vi "IMAQ FPGA Camera Link Line Builder (8 Tap U8 4X-1Y).vi"(8 "Input Valid In":bool=TRUE, 9 "Frame Valid In":bool, 10 "Line Valid In":bool, 11 "Pixel Data In":u8[](array[numeric])=[0, 0, 0, 0, 0, 0, 0, 0]) -> (0 "Output Valid":bool, 1 "Frame Valid Out":bool, 2 "Line Valid Out":bool, 3 "Pixel Bus x8 Out":cluster{"Pixels":u8[], "DV":bool[]}, 5 "Overflow":bool)   [LabVIEW 2017]
doc: "Camera Link cameras may return pixels from different parts of the image on each pixel clock. The Line Builder takes those pixels and combines them over multiple cycles to return a Pixel Bus of 8 pixels that are adjacent to each other. \n\nThis instance expects a camera with eigth taps (i.e. eight pixels returned on each pixel clock). The first two taps represents the left quarter of the image and the first valid pixels from these taps are located on the left of the image (pixels 0 and 1). The next two taps represents the next quarter of the image and the first valid pixels from these tap are located at Width/4, Width/4+1 of the image. The next two taps represents the next quarter of the image and the first valid pixels from these taps is located in the middle of the image (width/2 and width/2+1). The last two taps represent the last quarter of the image and the first valid pixels from these taps is located at 3/4*Width, and 3/4*Width +1 of the image."
uses:
  <vilib>/visionFPGA/Basics/Camera Link Acquisition/Controls/IMAQ FPGA Camera Link Line Builder State.ctl
  <vilib>/rvi/Emulation/niFpgaSctlEmulationGetInTimedLoop.vi
  <vilib>/Utility/error.llb/Clear Errors.vi
  <vilib>/rvi/DataTransferAndStorage/Container/Common/niFpgaContainerGetUniqueNameForEmu.vi
  <vilib>/rvi/DataTransferAndStorage/Container/Common/niFpgaContainerSetEmuInfo.vi
  <vilib>/rvi/eio/common/nirviEmuReportErrorAndStop.vi
  <vilib>/rvi/DataTransferAndStorage/Container/Common/niFpgaContainerExecOnDevCompGetState.vi
  <vilib>/rvi/Emulation/niFpgaEmulationIsFPGAContextNoSignature.vi
  <vilib>/rvi/Emulation/niFpgaProcessEmulError.vi
  <vilib>/rvi/errors/nirviReportUnexpectedCaseInternalError (U32).vi
  <vilib>/rvi/Memory/Memory_Emulation/niFpgaMemoryEmulationCacheClearOnFirstRun.vi
  <vilib>/rvi/Memory/Memory_Emulation/nirvimemoryEmulationManagerCache_MakeExclusive.vi
  <vilib>/rvi/Memory/Memory_Emulation/niFpgaMemoryEmulationValidateCache.vi
  <vilib>/rvi/Memory/Memory_Emulation/nirvimemoryEmulationManagerCache_InsertValue.vi
  <vilib>/rvi/Memory/Memory_Emulation/nirvimemoryEmulationManagerCache_ReleaseExclusive.vi
  <vilib>/rvi/Memory/Memory_Emulation/nirvimemoryEmulationManagerCache_GetValue.vi
  <vilib>/rvi/Memory/Memory_Emulation/nirvimemoryEmulationManagerCache_SetValue.vi
  <vilib>/rvi/Emulation/niFpgaSctlEmulationResourceMgr.vi
  <vilib>/rvi/LocalResourceManager/LocalResourceManager.xnode
  <vilib>/rvi/DataTransferAndStorage/Container/XNode/niFpgaContainer.xnode
  <vilib>/rvi/Memory/Memory_Emulation/niFpgaMemoryEmulationRefIn.vi
  <vilib>/visionFPGA/NI_VDM_FPGA_Basics.lvlib
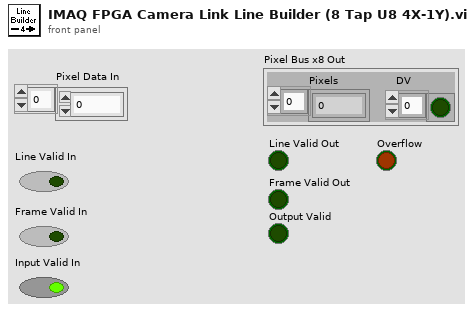
[diagram p1: front panel]
types:
  T1 = typedef "IMAQ FPGA Camera Link Line Builder State.ctl" = enum16{"Wait for First Valid Pixels", "Update Section 1", "Update Section 2", "Update Section 3", "Update Last Section", "Add Final Pack", "Add End of Line", "Check End of Image"}
  T2 = cluster{bool, u16, "Falling Edge":bool, bool, "Falling Edge":bool}
  T3 = cluster{bool, u16, "Falling Edge":bool, "Enum":T1, "Falling Edge":bool}
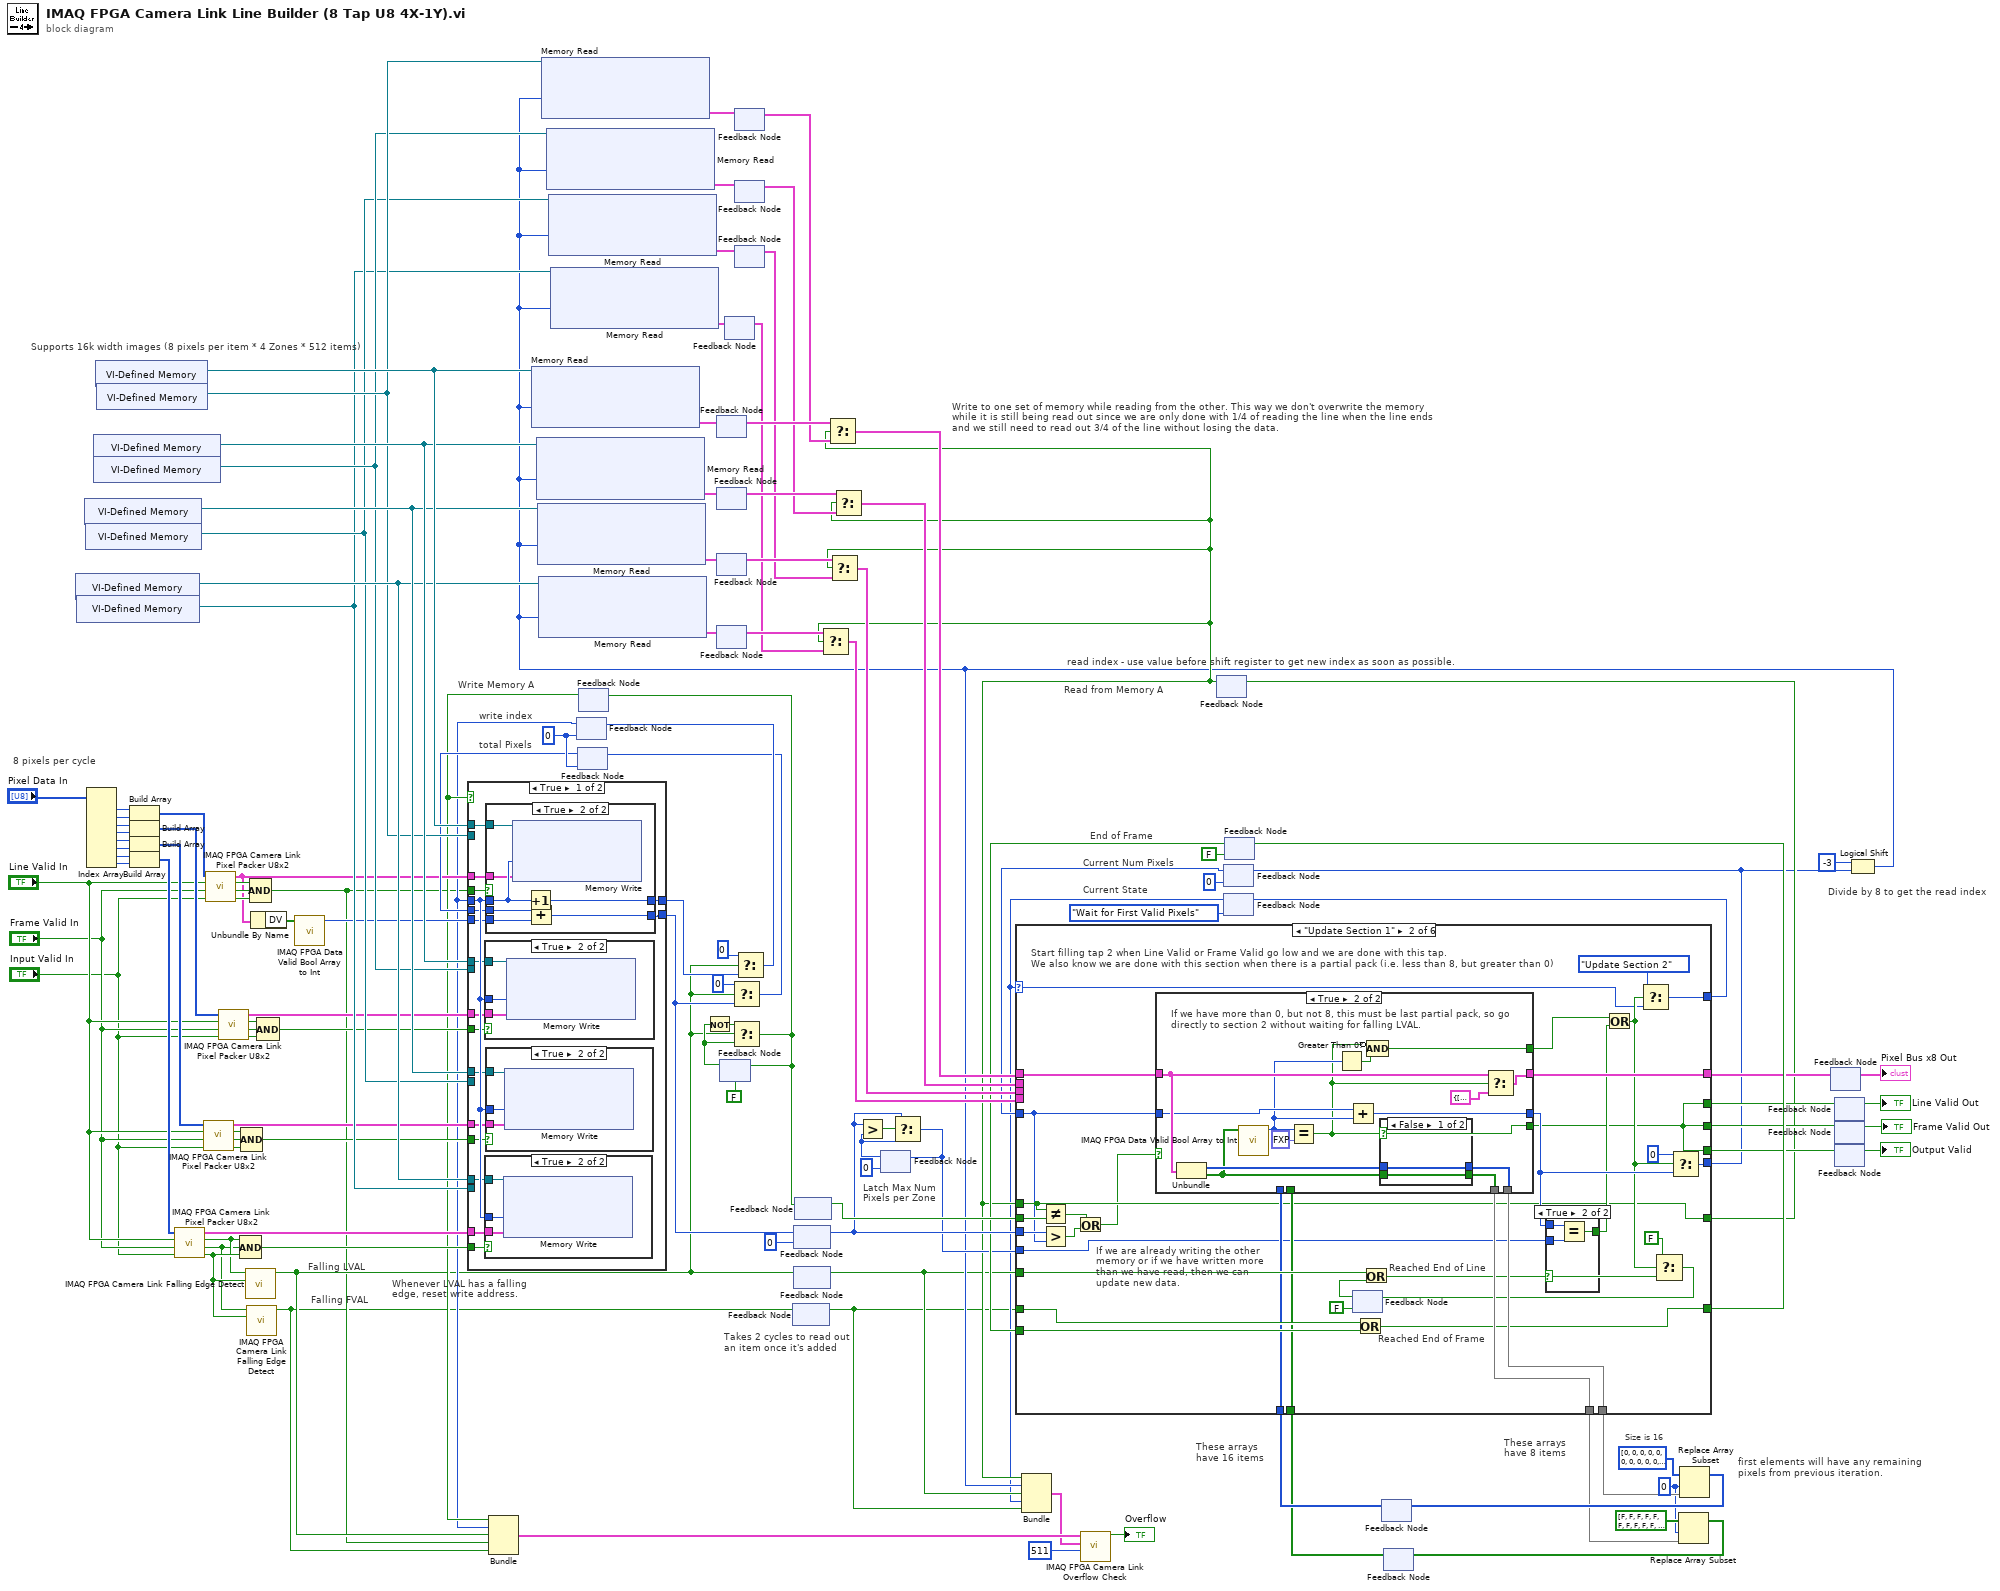
[diagram p0: block diagram]
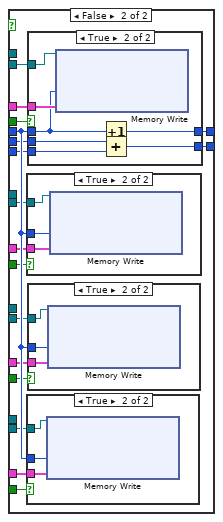
[diagram p6: hidden frame]
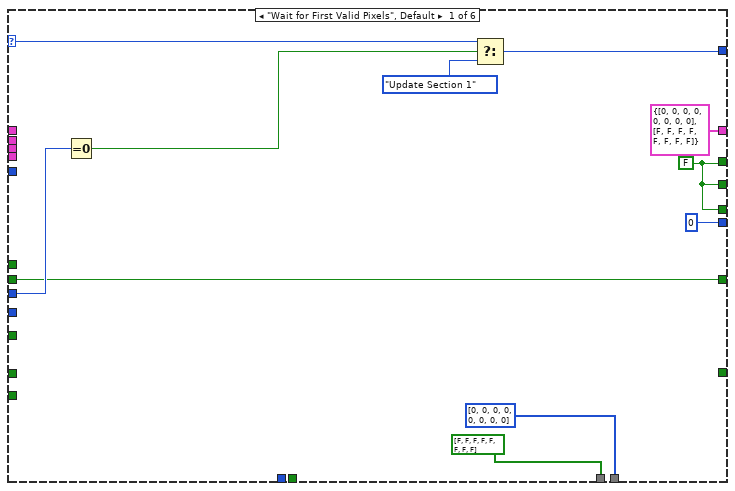
[diagram p11: hidden frame]
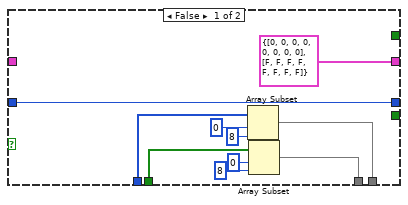
[diagram p12: hidden frame]
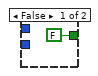
[diagram p14: hidden frame]
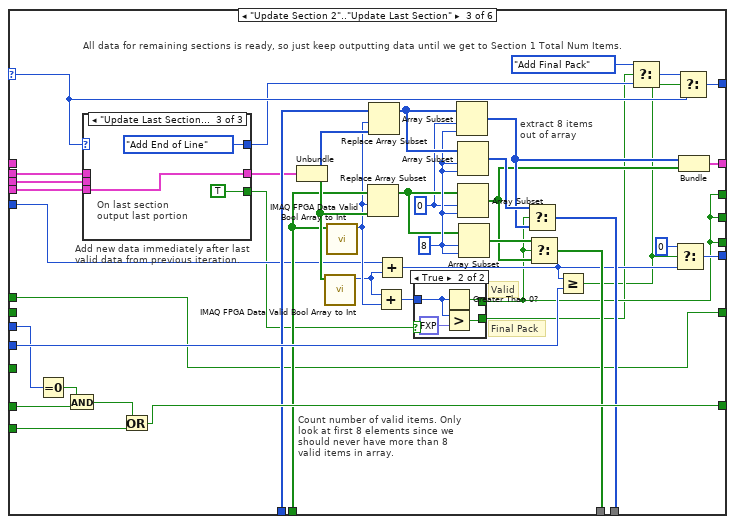
[diagram p15: hidden frame]
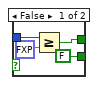
[diagram p16: hidden frame]
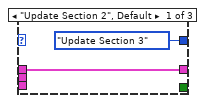
[diagram p17: hidden frame]
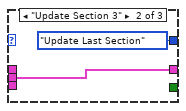
[diagram p18: hidden frame]
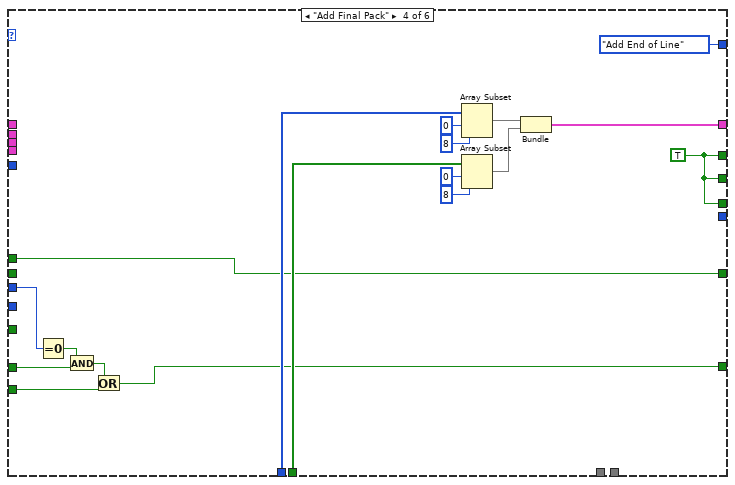
[diagram p19: hidden frame]
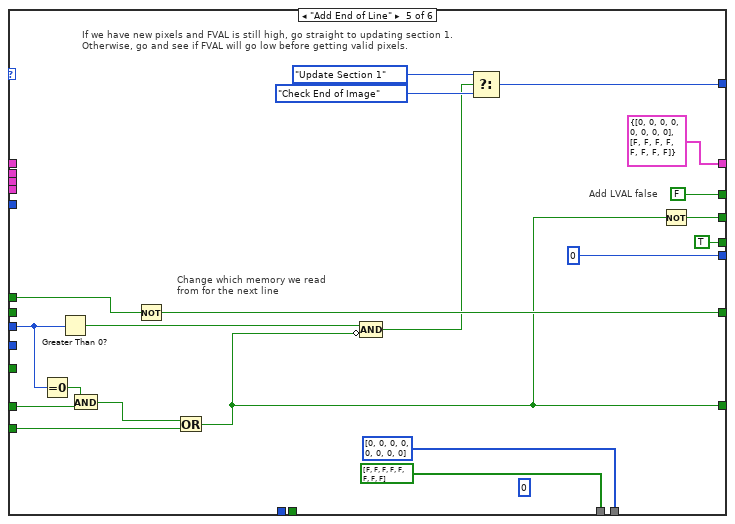
[diagram p20: hidden frame]
diagram:
  w41 = 0 ("index")
  w37 = u16 0
  # "Divide by 8 to get the read index"
  # "Latch Max Num Pixels per Zone"
  # "total Pixels"
  # "These arrays have 8 items"
  # "These arrays have 16 items"
  # "first elements will have any remaining pixels from previous iteration."
  # "Size is 16"
  # "Read from Memory A"
  # "Write Memory A"
  # "Write to one set of memory while reading from the other. This way we don't overwrite the memory while it is still being read out since we are only done with 1/4 of reading the line when the line ends and we still need to read out 3/4 of the line without losing the data."
  # "Falling FVAL"
  # "Falling LVAL"
  # "read index - use value before shift register to get new index as soon as possible."
  # "write index"
  # "Current State"
  # "End of Frame"
  # "Takes 2 cycles to read out an item once it's added"
  # "Current Num Pixels"
  # "Whenever LVAL has a falling edge, reset write address."
  # "Supports 16k width images (8 pixels per item * 4 Zones * 512 items)"
  # "8 pixels per cycle"
  n1 = xnode "VI-Defined Memory"() -> ("Memory Out"=w88:refnum<k21>)
  n2 = xnode "VI-Defined Memory"() -> ("Memory Out"=w80:refnum<k21>)
  n3 = xnode "VI-Defined Memory"() -> ("Memory Out"=w89:refnum<k21>)
  n4 = xnode "VI-Defined Memory"() -> ("Memory Out"=w81:refnum<k21>)
  n5 = Index Array(array="Pixel Data In") -> (element #1=w119:u8, element #2=w118:u8, element #3=w111:u8, element #4=w110:u8, element #5=w108:u8, element #6=w107:u8, element #7=w105:u8, element #8=w104:u8)  [unwired: 8 in]
  n6 = xnode "VI-Defined Memory"() -> ("Memory Out"=w90:refnum<k21>)
  n7 = xnode "VI-Defined Memory"() -> ("Memory Out"=w82:refnum<k21>)
  n8 = xnode "VI-Defined Memory"() -> ("Memory Out"=w91:refnum<k21>)
  n9 = xnode "VI-Defined Memory"() -> ("Memory Out"=w83:refnum<k21>)
  n10 = Build Array(w119, w118) -> (w117:u8[])
  n11 = Build Array(w111, w110) -> (w109:u8[])
  n12 = Build Array(w108, w107) -> (w106:u8[])
  n13 = Build Array(w105, w104) -> (w103:u8[])
  n14 = call <vilib>:"IMAQ FPGA Camera Link Pixel Packer U8x2.vi"("Input Valid"="Input Valid In", "Frame Valid In"="Frame Valid In", "Line Valid In"="Line Valid In", "Pixels In"=w103) -> ("Output Valid"=w30:bool, "Frame Valid Out"=w28:bool, "Line Valid Out"=w29:bool, "Pixel Bus x8 Out"=w65:cluster{"Pixels":u8[], "DV":bool[]})  [unwired: 4 in]
  n15 = call <vilib>:"IMAQ FPGA Camera Link Pixel Packer U8x2.vi"("Input Valid"="Input Valid In", "Frame Valid In"="Frame Valid In", "Line Valid In"="Line Valid In", "Pixels In"=w106) -> ("Output Valid"=w55:bool, "Frame Valid Out"=w56:bool, "Line Valid Out"=w57:bool, "Pixel Bus x8 Out"=w66:cluster{"Pixels":u8[], "DV":bool[]})  [unwired: 4 in]
  n16 = call <vilib>:"IMAQ FPGA Camera Link Pixel Packer U8x2.vi"("Input Valid"="Input Valid In", "Frame Valid In"="Frame Valid In", "Line Valid In"="Line Valid In", "Pixels In"=w117) -> ("Output Valid"=w114:bool, "Frame Valid Out"=w115:bool, "Line Valid Out"=w116:bool, "Pixel Bus x8 Out"=w31:cluster{"Pixels":u8[], "DV":bool[]})  [unwired: 4 in]
  n17 = call <vilib>:"IMAQ FPGA Camera Link Pixel Packer U8x2.vi"("Input Valid"="Input Valid In", "Frame Valid In"="Frame Valid In", "Line Valid In"="Line Valid In", "Pixels In"=w109) -> ("Output Valid"=w61:bool, "Frame Valid Out"=w60:bool, "Line Valid Out"=w59:bool, "Pixel Bus x8 Out"=w67:cluster{"Pixels":u8[], "DV":bool[]})  [unwired: 4 in]
  n18 = Compound Arithmetic op=AND(w29, w28, w30) -> (w53:bool)
  n19 = Compound Arithmetic op=AND(w57, w56, w55) -> (w54:bool)
  n20 = call <vilib>:"IMAQ FPGA Camera Link Falling Edge Detect.vi"("Input Valid"=w30, "Input"=w29) -> ("Falling Edge"=w12:bool)  [unwired: 9 in]
  n21 = call <vilib>:"IMAQ FPGA Camera Link Falling Edge Detect.vi"("Input Valid"=w30, "Input"=w28) -> ("Falling Edge"=w10:bool)  [unwired: 9 in]
  n22 = Compound Arithmetic op=AND(w116, w115, w114) -> (w11:bool)
  n23 = Unbundle By Name(w31) -> ("DV"=w40:bool[])
  n24 = Compound Arithmetic op=AND(w59, w60, w61) -> (w58:bool)
  n25 = call <vilib>:"IMAQ FPGA Data Valid Bool Array to Int.vi"("DV In"=w40) -> ("Sum DV Out"=w35:u8)  [unwired: 10 in]
  n26 = feedback #1(w37) -> (w13:u16)
  n27 = feedback #2(w37) -> (w36:u16)
  n28 = feedback #3() -> (w14:bool)  [unwired: 1 in]
  n29 = case shown="True" w14 {
    tunnel: [w142 w177] -> w120
    tunnel: w13 -> [w141 w176]
    tunnel: w11 -> [w132 w175]
    tunnel: w31 -> [w140 w174]
    tunnel: w67 -> [w139 w173]
    tunnel: w66 -> [w138 w172]
    tunnel: w65 -> [w137 w171]
    tunnel: w91 -> [w136 _]
    tunnel: w90 -> [w135 _]
    tunnel: w89 -> [w134 _]
    tunnel: w88 -> [w133 _]
    tunnel: w83 -> [_ w170]
    tunnel: w82 -> [_ w169]
    tunnel: w81 -> [_ w168]
    tunnel: w80 -> [_ w167]
    tunnel: w58 -> [w131 w166]
    tunnel: w54 -> [w130 w165]
    tunnel: w53 -> [w129 w164]
    tunnel: [w128 w163] -> w34
    tunnel: w36 -> [w127 w162]
    tunnel: w35 -> [w126 w161]
    frame True {
      n30 = case shown="True" w131 {
        tunnel: w139 -> [_ w150]
        tunnel: w135 -> [_ w151]
        tunnel: w141 -> [_ w149]
        frame False {
        }
        frame True {
          n31 = xnode ("Memory Write")("Address"=w149, "Data"=w150, "Memory In"=w151) -> ()  [unwired: 1 out]
        }
      }
      n32 = case shown="True" w129 {
        tunnel: w137 -> [_ w144]
        tunnel: w133 -> [_ w145]
        tunnel: w141 -> [_ w143]
        frame False {
        }
        frame True {
          n33 = xnode ("Memory Write")("Address"=w143, "Data"=w144, "Memory In"=w145) -> ()  [unwired: 1 out]
        }
      }
      n34 = case shown="True" w132 {
        tunnel: [w152 w154] -> w142
        tunnel: w141 -> [w153 w159]
        tunnel: w136 -> [_ w160]
        tunnel: w140 -> [_ w158]
        tunnel: [w153 w157] -> w128
        tunnel: w127 -> [w152 w156]
        tunnel: w126 -> [_ w155]
        frame False {
        }
        frame True {
          n35 = xnode ("Memory Write")("Address"=w159, "Data"=w158, "Memory In"=w160) -> ()  [unwired: 1 out]
          n36 = Increment(x=w159) -> (x+1=w157:u16)
          n37 = Add(x=w156, y=w155) -> (x+y=w154:u16)
        }
      }
      n38 = case shown="True" w130 {
        tunnel: w138 -> [_ w147]
        tunnel: w134 -> [_ w148]
        tunnel: w141 -> [_ w146]
        frame False {
        }
        frame True {
          n39 = xnode ("Memory Write")("Address"=w146, "Data"=w147, "Memory In"=w148) -> ()  [unwired: 1 out]
        }
      }
    }
    frame False {
      n40 = case shown="True" w166 {
        tunnel: w173 -> [_ w185]
        tunnel: w169 -> [_ w186]
        tunnel: w176 -> [_ w184]
        frame False {
        }
        frame True {
          n41 = xnode ("Memory Write")("Address"=w184, "Data"=w185, "Memory In"=w186) -> ()  [unwired: 1 out]
        }
      }
      n42 = case shown="True" w164 {
        tunnel: w171 -> [_ w179]
        tunnel: w167 -> [_ w180]
        tunnel: w176 -> [_ w178]
        frame False {
        }
        frame True {
          n43 = xnode ("Memory Write")("Address"=w178, "Data"=w179, "Memory In"=w180) -> ()  [unwired: 1 out]
        }
      }
      n44 = case shown="True" w175 {
        tunnel: [w187 w191] -> w177
        tunnel: w176 -> [w188 w193]
        tunnel: w170 -> [_ w195]
        tunnel: w174 -> [_ w194]
        tunnel: [w188 w192] -> w163
        tunnel: w162 -> [w187 w190]
        tunnel: w161 -> [_ w189]
        frame False {
        }
        frame True {
          n45 = xnode ("Memory Write")("Address"=w193, "Data"=w194, "Memory In"=w195) -> ()  [unwired: 1 out]
          n46 = Increment(x=w193) -> (x+1=w192:u16)
          n47 = Add(x=w190, y=w189) -> (x+y=w191:u16)
        }
      }
      n48 = case shown="True" w165 {
        tunnel: w172 -> [_ w182]
        tunnel: w168 -> [_ w183]
        tunnel: w176 -> [_ w181]
        frame False {
        }
        frame True {
          n49 = xnode ("Memory Write")("Address"=w181, "Data"=w182, "Memory In"=w183) -> ()  [unwired: 1 out]
        }
      }
    }
  }
  n50 = Bundle(w14, w13, "Falling Edge"=w12, w11, "Falling Edge"=w10) -> (w9:T2)  [unwired: 1 in]
  n51 = feedback #4() -> (w75:cluster{"Pixels":u8[], "DV":bool[]})  [unwired: 1 in]
  n52 = feedback #5() -> (w73:cluster{"Pixels":u8[], "DV":bool[]})  [unwired: 1 in]
  n53 = feedback #6() -> (w71:cluster{"Pixels":u8[], "DV":bool[]})  [unwired: 1 in]
  n54 = feedback #7() -> (w69:cluster{"Pixels":u8[], "DV":bool[]})  [unwired: 1 in]
  n55 = feedback #8(FALSE) -> (w39:bool)
  n56 = Not(x=w39) -> (.not. x?=w112:bool)
  n57 = feedback #9() -> (w68:cluster{"Pixels":u8[], "DV":bool[]})  [unwired: 1 in]
  n58 = Select(t=u16 0, s=w12, f=w120) -> (s? t:f=w32:u16)
  n59 = feedback-in #2(w32) -> ()
  n60 = Select(t=w112, s=w12, f=w39) -> (s? t:f=w27:bool)
  n61 = feedback-in #3(w27) -> ()
  n62 = feedback-in #8(w27) -> ()
  n63 = feedback #10() -> (w74:cluster{"Pixels":u8[], "DV":bool[]})  [unwired: 1 in]
  n64 = feedback #11() -> (w72:cluster{"Pixels":u8[], "DV":bool[]})  [unwired: 1 in]
  n65 = feedback #12() -> (w70:cluster{"Pixels":u8[], "DV":bool[]})  [unwired: 1 in]
  n66 = Select(t=u16 0, s=w12, f=w34) -> (s? t:f=w33:u16)
  n67 = feedback-in #1(w33) -> ()
  n68 = feedback #13() -> (w3:bool)  [unwired: 1 in]
  n69 = feedback-in #13(w10) -> ()
  n70 = feedback-in #14(w120) -> ()
  n71 = feedback #14(u16 0) -> (w25:u16)
  n72 = feedback-in #15(w12) -> ()
  n73 = feedback #15() -> (w6:bool)  [unwired: 1 in]
  n74 = feedback #16() -> (w45:bool)  [unwired: 1 in]
  n75 = feedback-in #16(w27) -> ()
  n76 = feedback #17(u16 0) -> (w24:u16)
  n77 = Greater?(x=w25, y=w24) -> (0:w26:bool)
  n78 = Select(t=w25, s=w26, f=w24) -> (s? t:f=w15:u16)
  n79 = feedback-in #17(w15) -> ()
  n80 = feedback #18() -> (w8:bool)  [unwired: 1 in]
  n81 = Select(t=w69, s=w8, f=w68) -> (s? t:f=w62:cluster{"Pixels":u8[], "DV":bool[]})
  n82 = Select(t=w75, s=w8, f=w74) -> (s? t:f=w44:cluster{"Pixels":u8[], "DV":bool[]})
  n83 = Select(t=w71, s=w8, f=w70) -> (s? t:f=w63:cluster{"Pixels":u8[], "DV":bool[]})
  n84 = Select(t=w73, s=w8, f=w72) -> (s? t:f=w64:cluster{"Pixels":u8[], "DV":bool[]})
  n85 = feedback #19(u16 0) -> (w17:u16)
  n86 = feedback #20(IMAQ_FPGA_Camera_Link_Line_Builder_State."Wait for First Valid Pixels" ("Enum")) -> (w4:T1)
  n87 = feedback #21(FALSE) -> (w19:bool)
  n88 = feedback #22() -> (w43:u8[])  [unwired: 1 in]
  n89 = feedback #23() -> (w42:bool[])  [unwired: 1 in]
  n90 = case shown="\"Update Section 1\"" w4 {
    selector: w4 -> [w206 w207 w298 _ _ w385]
    tunnel: [w205 w239 w312 IMAQ_FPGA_Camera_Link_Line_Builder_State."Add End of Line" ("Enum") w360 w386] -> w16
    tunnel: w6 -> [_ w237 _ _ _ _]
    tunnel: w3 -> [_ w233 w278 w329 w349 w372]
    tunnel: [u16 0 w236 w308 _ u16 0 u16 0] -> w22
    tunnel: w17 -> [_ w213 w285 _ _ _]
    tunnel: w25 -> [w201 w214 w279 w330 w350 w373]
    tunnel: w15 -> [_ w226 w309 _ _ _]
    tunnel: [_ w229 w310 w332 w346 w382] -> w121
    tunnel: w19 -> [_ w234 w311 w333 w364 w388]
    tunnel: w44 -> [_ w223 _ _ _ _]
    tunnel: w64 -> [_ _ w300 _ _ _]
    tunnel: w63 -> [_ _ w297 _ _ _]
    tunnel: w62 -> [_ _ w296 _ _ _]
    tunnel: w45 -> [w200 w216 _ _ _ w369]
    tunnel: [w200 w217 w272 w334 w355 w368] -> w46
    tunnel: w8 -> [_ w217 w272 w334 w356 w368]
    tunnel: w42 -> [_ w227 w295 w337 _ _]
    tunnel: w43 -> [_ w228 w304 w338 _ _]
    tunnel: [cluster{"Pixels":u8[], "DV":bool[]} {"Pixels"=[0, 0, 0, 0, 0, 0, 0, 0], "DV"=[FALSE, FALSE, FALSE, FALSE, FALSE, FALSE, FALSE, FALSE]} ("Data") w232 w307 w336 cluster{"Pixels":u8[], "DV":bool[]} {"Pixels"=[0, 0, 0, 0, 0, 0, 0, 0], "DV"=[FALSE, FALSE, FALSE, FALSE, FALSE, FALSE, FALSE, FALSE]} ("Data") cluster{"Pixels":u8[], "DV":bool[]} {"Pixels"=[0, 0, 0, 0, 0, 0, 0, 0], "DV"=[FALSE, FALSE, FALSE, FALSE, FALSE, FALSE, FALSE, FALSE]} ("Data")] -> w99
    tunnel: [w196 w210 w275 w335 FALSE FALSE] -> w97
    tunnel: [w196 w210 w275 w335 w357 w378] -> w96
    tunnel: [w196 w210 w275 w335 TRUE TRUE] -> w95
    tunnel: [bool[] [FALSE, FALSE, FALSE, FALSE, FALSE, FALSE, FALSE, FALSE] ("DV") w231 w289 _ bool[] [FALSE, FALSE, FALSE, FALSE, FALSE, FALSE, FALSE, FALSE] bool[] [FALSE, FALSE, FALSE, FALSE, FALSE, FALSE, FALSE, FALSE]] -> w47
    tunnel: [u8[] [0, 0, 0, 0, 0, 0, 0, 0] ("Pixels") w230 w288 _ u8[] [0, 0, 0, 0, 0, 0, 0, 0] ("Pixels") u8[] [0, 0, 0, 0, 0, 0, 0, 0] ("Pixels")] -> w48
    frame "Wait for First Valid Pixels", Default {
      w196 = FALSE
      n91 = Equal To 0?(x=w201) -> (x = 0?=w204:bool)
      n92 = Select(t=w206, s=w204, f=IMAQ_FPGA_Camera_Link_Line_Builder_State."Update Section 1") -> (s? t:f=w205:T1)
    }
    frame "Update Section 1" {
      # "If we are already writing the other memory or if we have written more than we have read, then we can update new data."
      # "Reached End of Frame"
      # "Reached End of Line"
      # "Start filling tap 2 when Line Valid or Frame Valid go low and we are done with this tap.\nWe also know we are done with this section when there is a partial pack (i.e. less than 8, but greater than 0)"
      n93 = Not Equal?(x=w217, y=w216) -> (x != y?=w215:bool)
      n94 = Greater?(x=w214, y=w213) -> (0:w212:bool)
      n95 = Or(x=w215, y=w212) -> (x .or. y?=w211:bool)
      n96 = case shown="True" w211 {
        tunnel: w223 -> [_ w260]
        tunnel: w213 -> [w249 w258]
        tunnel: [w249 w263] -> w235
        tunnel: [cluster{"Pixels":u8[], bool[]} {"Pixels"=[0, 0, 0, 0, 0, 0, 0, 0], [FALSE, FALSE, FALSE, FALSE, FALSE, FALSE, FALSE, FALSE]} w262] -> w232
        tunnel: [w240 w253] -> w231
        tunnel: [w244 w254] -> w230
        tunnel: w228 -> [w247 _]
        tunnel: w227 -> [w243 _]
        tunnel: [_ w252] -> w210
        tunnel: [_ w250] -> w209
        frame False {
          n97 = Array Subset(array=w247, index=0, length=8) -> (w244:u8[])
          n98 = Array Subset(array=w243, index=0, length=8) -> (w240:bool[])
        }
        frame True {
          # "If we have more than 0, but not 8, this must be last partial pack, so go directly to section 2 without waiting for falling LVAL."
          n99 = Unbundle(w260) -> ("Pixels"=w256:u8[], "DV"=w255:bool[])
          n100 = call <vilib>:"IMAQ FPGA Data Valid Bool Array to Int.vi"("DV In"=w255) -> ("Sum DV Out"=w257:u8)  [unwired: 10 in]
          n101 = Equal?(x=w257, y=fxp<+,4,4> 8.0) -> (x = y?=w252:bool)
          n102 = Greater Than 0?(x=w257) -> (x > 0?=w251:bool)
          n103 = Add(x=w258, y=w257) -> (x+y=w263:u16)
          n104 = Compound Arithmetic op=AND(invert w252, w251) -> (w250:bool)
          n105 = case shown="False" w252 {
            tunnel: w256 -> [w265 _]
            tunnel: w255 -> [w264 _]
            tunnel: [w265 _] -> w254
            tunnel: [w264 _] -> w253
            frame False {
            }
            frame True {
            }
          }
          n106 = Select(t=w260, s=w252, f=cluster{"Pixels":u8[], "DV":bool[]} {"Pixels"=[0, 0, 0, 0, 0, 0, 0, 0], "DV"=[FALSE, FALSE, FALSE, FALSE, FALSE, FALSE, FALSE, FALSE]}) -> (s? t:f=w262:cluster{"Pixels":u8[], "DV":bool[]})
        }
      }
      n107 = feedback #24(FALSE) -> (w222:bool)
      n108 = Or(x=w233, y=w234) -> (x .or. y?=w229:bool)
      n109 = Or(x=w237, y=w222) -> (x .or. y?=w221:bool)
      n110 = case shown="True" w221 {
        tunnel: w226 -> [_ w268]
        tunnel: w235 -> [_ w269]
        tunnel: [FALSE w267] -> w224
        frame False {
        }
        frame True {
          n111 = Equal?(x=w269, y=w268) -> (x = y?=w267:bool)
        }
      }
      n112 = Or(x=w209, y=w224) -> (x .or. y?=w220:bool)
      n113 = Select(t=IMAQ_FPGA_Camera_Link_Line_Builder_State."Update Section 2" ("Enum"), s=w220, f=w207) -> (s? t:f=w239:T1)
      n114 = Select(t=FALSE, s=w220, f=w221) -> (s? t:f=w218:bool)
      n115 = feedback-in #24(w218) -> ()
      n116 = Select(t=u16 0, s=w220, f=w235) -> (s? t:f=w236:u16)
    }
    frame "Update Section 2".."Update Last Section" {
      w287 = 0 ("index")
      w302 = 8 ("length")
      # "Final Pack"
      # "Valid"
      # "extract 8 items out of array"
      # "Add new data immediately after last valid data from previous iteration."
      # "Count number of valid items. Only look at first 8 elements since we should never have more than 8 valid items in array."
      # "All data for remaining sections is ready, so just keep outputting data until we get to Section 1 Total Num Items."
      n117 = Equal To 0?(x=w279) -> (x = 0?=w280:bool)
      n118 = And(x=w280, y=w278) -> (x .and. y?=w277:bool)
      n119 = case shown="\"Update Last Section\"" w298 {
        tunnel: w300 -> [w322 _ _]
        tunnel: [w322 w323 w326] -> w299
        tunnel: [IMAQ_FPGA_Camera_Link_Line_Builder_State."Update Section 3" ("t") IMAQ_FPGA_Camera_Link_Line_Builder_State."Update Last Section" ("t") IMAQ_FPGA_Camera_Link_Line_Builder_State."Add End of Line" ("t")] -> w283
        tunnel: w297 -> [_ w323 _]
        tunnel: w296 -> [_ _ w326]
        tunnel: [_ _ TRUE] -> w276
        frame "Update Section 2", Default {
        }
        frame "Update Section 3" {
        }
        frame "Update Last Section" {
          # "On last section output last portion"
        }
      }
      n120 = Or(x=w277, y=w311) -> (x .or. y?=w310:bool)
      n121 = Unbundle(w299) -> ("Pixels"=w306:u8[], "DV"=w305:bool[])
      n122 = call <vilib>:"IMAQ FPGA Data Valid Bool Array to Int.vi"("DV In"=w305) -> ("Sum DV Out"=w284:u8)  [unwired: 10 in]
      n123 = call <vilib>:"IMAQ FPGA Data Valid Bool Array to Int.vi"("DV In"=w295) -> ("Sum DV Out"=w294:u8)  [unwired: 10 in]
      n124 = Replace Array Subset(array=w295, new element=w305, index=w294) -> (w301:bool[])
      n125 = Replace Array Subset(array=w304, new element=w306, index=w294) -> (w303:u8[])
      n126 = Add(x=w284, y=w294) -> (x+y=w273:u8)
      n127 = Add(x=w285, y=w284) -> (x+y=w286:u16)
      n128 = case shown="True" w276 {
        tunnel: [w316 w320] -> w275
        tunnel: [FALSE w318] -> w274
        tunnel: w273 -> [w313 w317]
        frame False {
          n129 = Greater Or Equal?(x=w313, y=fxp<+,5,5> 8.0) -> (x >= y?=w316:bool)
        }
        frame True {
          n130 = Greater Than 0?(x=w317) -> (x > 0?=w320:bool)
          n131 = Greater?(x=w317, y=fxp<+,5,5> 8.0) -> (0:w318:bool)
        }
      }
      n132 = Array Subset(array=w303, index=w287, length=w302) -> (w292:u8[])
      n133 = Array Subset(array=w303, index=w302, length=w302) -> (w293:u8[])
      n134 = Array Subset(array=w301, index=w287, length=w302) -> (w290:bool[])
      n135 = Array Subset(array=w301, index=w302, length=w302) -> (w291:bool[])
      n136 = Select(t=w293, s=w275, f=w292) -> (s? t:f=w288:u8[])
      n137 = Select(t=w291, s=w275, f=w290) -> (s? t:f=w289:bool[])
      n138 = Greater Or Equal?(x=w286, y=w309) -> (x >= y?=w271:bool)
      n139 = Select(t=IMAQ_FPGA_Camera_Link_Line_Builder_State."Add Final Pack", s=w274, f=w283) -> (s? t:f=w282:T1)
      n140 = Select(t=u16 0, s=w271, f=w286) -> (s? t:f=w308:u16)
      n141 = Select(t=w282, s=w271, f=w298) -> (s? t:f=w312:T1)
      n142 = Bundle(w292, w290) -> (w307:cluster{u8[], bool[]})  [unwired: 1 in]
    }
    frame "Add Final Pack" {
      w335 = TRUE
      n143 = Equal To 0?(x=w330) -> (x = 0?=w331:bool)
      n144 = And(x=w331, y=w329) -> (x .and. y?=w328:bool)
      n145 = Or(x=w328, y=w333) -> (x .or. y?=w332:bool)
      n146 = Array Subset(array=w338, index=0, length=8) -> (w340:u8[])
      n147 = Array Subset(array=w337, index=0, length=8) -> (w339:bool[])
      n148 = Bundle(w340, w339) -> (w336:cluster{u8[], bool[]})  [unwired: 1 in]
    }
    frame "Add End of Line" {
      (unwired) i8 0
      # "Change which memory we read from for the next line"
      # "Add LVAL false"
      # "If we have new pixels and FVAL is still high, go straight to updating section 1. Otherwise, go and see if FVAL will go low before getting valid pixels."
      n149 = Equal To 0?(x=w350) -> (x = 0?=w351:bool)
      n150 = Greater Than 0?(x=w350) -> (x > 0?=w363:bool)
      n151 = And(x=w351, y=w349) -> (x .and. y?=w348:bool)
      n152 = Not(x=w356) -> (.not. x?=w355:bool)
      n153 = Or(x=w348, y=w364) -> (x .or. y?=w346:bool)
      n154 = Compound Arithmetic op=AND(w363, invert w346) -> (w347:bool)
      n155 = Select(t=IMAQ_FPGA_Camera_Link_Line_Builder_State."Update Section 1" ("Enum"), s=w347, f=IMAQ_FPGA_Camera_Link_Line_Builder_State."Check End of Image" ("Enum")) -> (s? t:f=w360:T1)
      n156 = Not(x=w346) -> (.not. x?=w357:bool)
    }
    frame "Check End of Image" {
      # "If not reading from same memory or there's already data, go straight to Updating Section 1."
      # "Stay in this state until we get new pixels, or we get end of image"
      # "End of Image"
      n157 = Equal To 0?(x=w373) -> (x = 0?=w374:bool)
      n158 = Greater Than 0?(x=w373) -> (x > 0?=w370:bool)
      n159 = Not Equal?(x=w368, y=w369) -> (x != y?=w367:bool)
      n160 = And(x=w374, y=w372) -> (x .and. y?=w371:bool)
      n161 = Or(x=w367, y=w370) -> (x .or. y?=w366:bool)
      n162 = Or(x=w371, y=w388) -> (x .or. y?=w379:bool)
      n163 = Select(t=IMAQ_FPGA_Camera_Link_Line_Builder_State."Update Section 1" ("Enum"), s=w366, f=IMAQ_FPGA_Camera_Link_Line_Builder_State."Wait for First Valid Pixels" ("Enum")) -> (s? t:f=w387:T1)
      n164 = Or(x=w366, y=w379) -> (x .or. y?=w384:bool)
      n165 = Select(t=w387, s=w384, f=w385) -> (s? t:f=w386:T1)
      n166 = Select(t=FALSE, s=w384, f=w379) -> (s? t:f=w382:bool)
      n167 = Not(x=w379) -> (.not. x?=w378:bool)
    }
  }
  n168 = feedback-in #18(w46) -> ()
  n169 = feedback-in #19(w22) -> ()
  n170 = feedback-in #20(w16) -> ()
  n171 = feedback-in #21(w121) -> ()
  n172 = Replace Array Subset(array=bool[] [FALSE, FALSE, FALSE, FALSE, FALSE, FALSE, FALSE, FALSE, FALSE, FALSE, FALSE, FALSE, FALSE, FALSE, FALSE, FALSE], new element=w47, index=w41) -> (w49:bool[])
  n173 = feedback-in #23(w49) -> ()
  n174 = Replace Array Subset(array=u8[] [0, 0, 0, 0, 0, 0, 0, 0, 0, 0, 0, 0, 0, 0, 0, 0] ("Pixels"), new element=w48, index=w41) -> (w51:u8[])
  n175 = feedback-in #22(w51) -> ()
  n176 = feedback #25() -> (→"Pixel Bus x8 Out":cluster{"Pixels":u8[], "DV":bool[]})  [unwired: 1 in]
  n177 = feedback-in #25(w99) -> ()
  n178 = feedback #26() -> (→"Line Valid Out":bool)  [unwired: 1 in]
  n179 = feedback-in #26(w97) -> ()
  n180 = feedback #27() -> (→"Frame Valid Out":bool)  [unwired: 1 in]
  n181 = feedback-in #27(w96) -> ()
  n182 = feedback #28() -> (→"Output Valid":bool)  [unwired: 1 in]
  n183 = feedback-in #28(w95) -> ()
  n184 = Logical Shift(y=i16 -3, x=w22) -> (x << y=w7:u16)
  n185 = xnode ("Memory Read")("Address"=w7, "Memory In"=w91) -> ("Data"=w87:cluster{"Pixels":u8[], "DV":bool[]})  [unwired: 1 out]
  n186 = xnode ("Memory Read")("Address"=w7, "Memory In"=w90) -> ("Data"=w86:cluster{"Pixels":u8[], "DV":bool[]})  [unwired: 1 out]
  n187 = xnode ("Memory Read")("Address"=w7, "Memory In"=w89) -> ("Data"=w85:cluster{"Pixels":u8[], "DV":bool[]})  [unwired: 1 out]
  n188 = xnode ("Memory Read")("Address"=w7, "Memory In"=w88) -> ("Data"=w84:cluster{"Pixels":u8[], "DV":bool[]})  [unwired: 1 out]
  n189 = xnode ("Memory Read")("Address"=w7, "Memory In"=w83) -> ("Data"=w76:cluster{"Pixels":u8[], "DV":bool[]})  [unwired: 1 out]
  n190 = xnode ("Memory Read")("Address"=w7, "Memory In"=w82) -> ("Data"=w77:cluster{"Pixels":u8[], "DV":bool[]})  [unwired: 1 out]
  n191 = xnode ("Memory Read")("Address"=w7, "Memory In"=w81) -> ("Data"=w78:cluster{"Pixels":u8[], "DV":bool[]})  [unwired: 1 out]
  n192 = xnode ("Memory Read")("Address"=w7, "Memory In"=w80) -> ("Data"=w79:cluster{"Pixels":u8[], "DV":bool[]})  [unwired: 1 out]
  n193 = feedback-in #4(w87) -> ()
  n194 = feedback-in #5(w86) -> ()
  n195 = feedback-in #6(w85) -> ()
  n196 = feedback-in #7(w84) -> ()
  n197 = feedback-in #9(w79) -> ()
  n198 = feedback-in #10(w76) -> ()
  n199 = feedback-in #11(w77) -> ()
  n200 = feedback-in #12(w78) -> ()
  n201 = Bundle(w8, w7, "Falling Edge"=w6, "Enum"=w4, "Falling Edge"=w3) -> (w5:T3)  [unwired: 1 in]
  n202 = call <vilib>:"IMAQ FPGA Camera Link Overflow Check.vi"("Max Index"=u16 511, "Read Info"=w5, "Write Info"=w9) -> ("Overlfow"=→"Overflow":bool)  [unwired: 8 in]
